vi "SortVisuualizationModuleInfoArray.vi"(11 "Open Visualization VIs in":T1[](array[typedef])) -> (3 "Array":T1[](array[typedef]))   [LabVIEW 2018]
uses:
  OpenVisualizationVIs.ctl
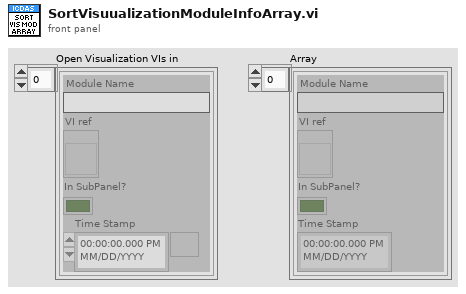
[diagram p1: front panel]
types:
  T1 = typedef "OpenVisualizationVIs.ctl" = cluster{"Module Name":string, "VI ref":refnum<vi>, "In SubPanel?":bool, "Time Stamp":timestamp}
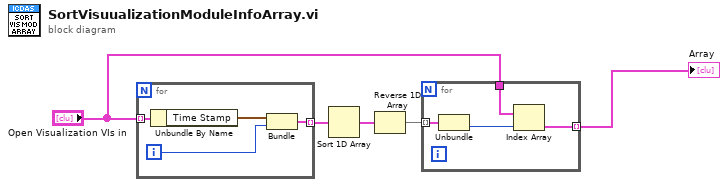
[diagram p0: block diagram]
diagram:
  n1 = for {
    tunnel: "Open Visualization VIs in" -> [w9] mode=indexing
    tunnel: [w6] -> w1 mode=indexing
    i -> [w7]
    n2 = Unbundle By Name(w9) -> ("Time Stamp"=w8:timestamp)
    n3 = Bundle("Time Stamp"=w8, w7) -> (w6:cluster{"Time Stamp":timestamp, i32})  [unwired: 1 in]
  }
  n4 = Sort 1D Array(array=w1) -> (sorted array=w2:cluster{"Time Stamp":timestamp, i32}[])
  n5 = Reverse 1D Array(array=w2) -> (reversed array=w3:cluster{"Time Stamp":timestamp, i32}[])
  n6 = for {
    tunnel: w3 -> [w13] mode=indexing
    tunnel: "Open Visualization VIs in" -> [w12]
    tunnel: [w10] -> w5 mode=indexing
    n7 = Unbundle(w13) -> (w11:i32)  [unwired: 1 out]
    n8 = Index Array(array=w12, index=w11) -> (element=w10:T1)
  }
  "Array" <- w5
